vi "AlliGator Enter CV Analysis Parameters Dialog.vi"(8 "Error In":errorcluster) -> (0 "Error Out":errorcluster, 1 "Cancelled?":bool, 3 "Function Parameters out":T1={"Function"=enum."Single-Exponential", "Amplitude"=0.0, "Exponent/Scale"=0.0, "Baseline"=0.0, "Residuals SDV"=0.0, "Minimum CL (%)"=1.0, "Analysis Type"=enum."Reference", "Bootstrap SDV x Scale Factor"=1.0, "Residuals SDV x Scale Factor"=1.0, "Low CL Percentile to Reject (%)"=1.0} {"Low CL Percentile to Reject (%)" min=0.0 max=100.0; "Residuals SDV x Scale Factor" min=0.0 max=100.0; "Bootstrap SDV x Scale Factor" min=0.0 max=100.0; "Minimum CL (%)" min=1.0})   [LabVIEW 2021, in "AlliGator Decay Fit Parameter Map.lvlib"]
doc: "Lets the user enter the power law parameters describing the CV_tau(I) dependency, where <B>I</B> is the pixel intensity and <B>CV_tau</B> is the lifetime coefficient of variation obtained from calibration measurements."
uses:
  AlliGator Decay Fit Parameter Map.lvlib
  AlliGator Function Parameters.ctl
  AlliGator CV(tau) Model Function.ctl
  Lifetime & Other Parameters/AlliGator Lifetime & Other Parameters.lvlib
panel:
  in  "Function Parameters":T1={"Function"=enum."Single-Exponential", "Amplitude"=0.0, "Exponent/Scale"=0.0, "Baseline"=0.0, "Residuals SDV"=0.0, "Minimum CL (%)"=1.0, "Analysis Type"=enum."Reference", "Bootstrap SDV x Scale Factor"=1.0, "Residuals SDV x Scale Factor"=1.0, "Low CL Percentile to Reject (%)"=1.0} {"Low CL Percentile to Reject (%)" min=0.0 max=100.0; "Residuals SDV x Scale Factor" min=0.0 max=100.0; "Bootstrap SDV x Scale Factor" min=0.0 max=100.0; "Minimum CL (%)" min=0.0 max=100.0}
  out "Message":string
  in  "Cancel":bool
  in  "OK":bool
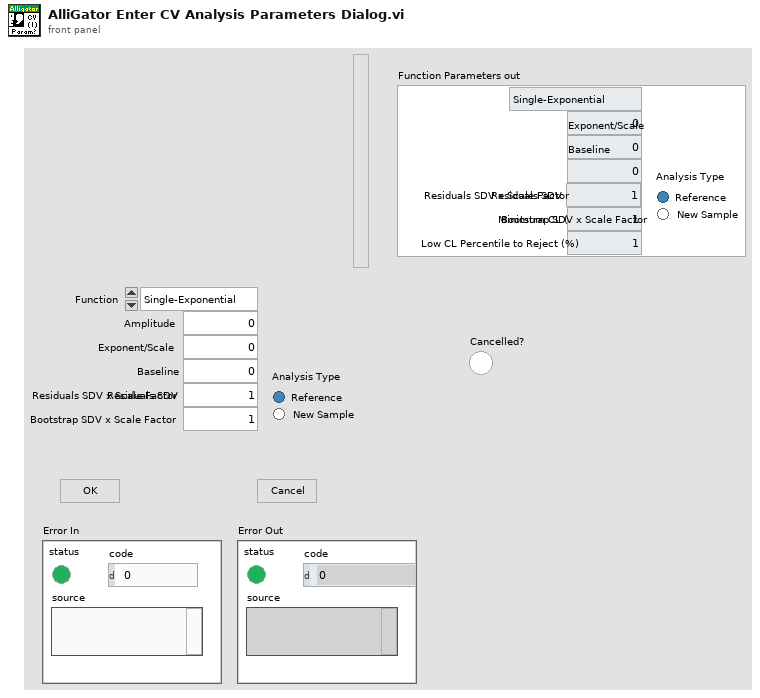
[diagram p1: front panel]
types:
  T1 = typedef "AlliGator Decay Fit Parameter Map.lvlib/AlliGator Function Parameters.ctl" = cluster{"Function":T2, "Amplitude":dbl, "Exponent/Scale":dbl, "Baseline":dbl, "Residuals SDV":dbl, "Minimum CL (%)":dbl, "Analysis Type":enum32{"Reference", "New Sample"}, "Bootstrap SDV x Scale Factor":dbl, "Residuals SDV x Scale Factor":dbl, "Low CL Percentile to Reject (%)":dbl}
  T2 = typedef "AlliGator Lifetime & Other Parameters.lvlib/AlliGator CV(tau) Model Function.ctl" = enum16{"Single-Exponential", "Power Law"}
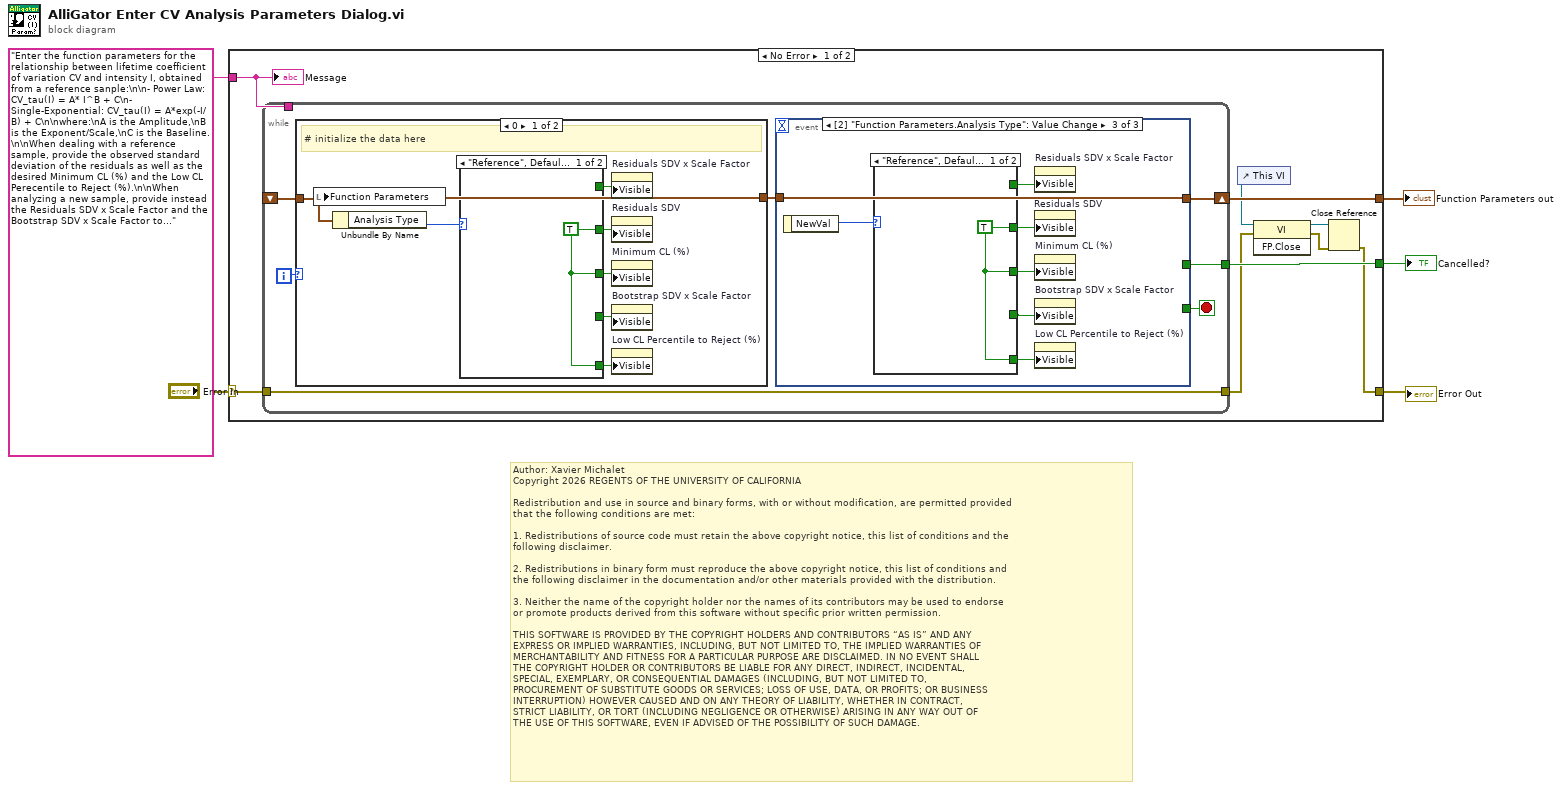
[diagram p0: block diagram]
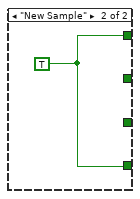
[diagram p2: hidden frame]
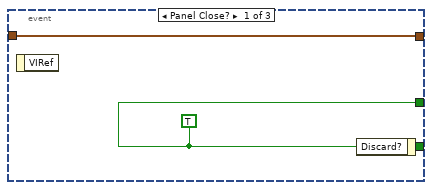
[diagram p4: hidden frame]
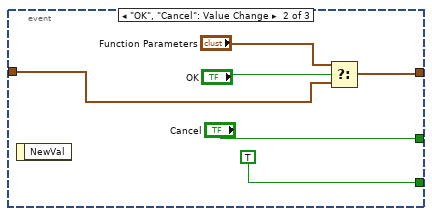
[diagram p5: hidden frame]
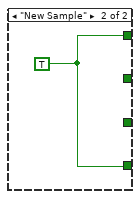
[diagram p6: hidden frame]
diagram:
  # "Author: Xavier Michalet\nCopyright 2026 REGENTS OF THE UNIVERSITY OF CALIFORNIA\n\nRedistribution and use in source and binary forms, with or without modification, are permitted provided\nthat the following conditions are met:\n\n1. Redistributions of source code must retain the above copyright notice, this list of conditions and the\nfollowing disclaimer.\n\n2. Redistributions in binary form must reproduce the above copyright notice, this list of conditions and\nthe following disclaimer in the documentation and/or other materials provided with the distribution.\n\n3. Neither the name of the copyright holder nor the names of its contributors may be used to endorse \nor promote products derived from this software without specific prior written permission.\n\nTHIS SOFTWARE IS PROVIDED BY THE COPYRIGHT HOLDERS AND CONTRIBUTORS “AS IS” AND ANY \nEXPRESS OR IMPLIED WARRANTIES, INCLUDING, BUT NOT LIMITED TO, THE IMPLIED WARRANTIES OF\nMERCHANTABILITY AND FITNESS FOR A PARTICULAR PURPOSE ARE DISCLAIMED. IN NO EVENT SHALL\nTHE COPYRIGHT HOLDER OR CONTRIBUTORS BE LIABLE FOR ANY DIRECT, INDIRECT, INCIDENTAL, \nSPECIAL, EXEMPLARY, OR CONSEQUENTIAL DAMAGES (INCLUDING, BUT NOT LIMITED TO, \nPROCUREMENT OF SUBSTITUTE GOODS OR SERVICES; LOSS OF USE, DATA, OR PROFITS; OR BUSINESS\nINTERRUPTION) HOWEVER CAUSED AND ON ANY THEORY OF LIABILITY, WHETHER IN CONTRACT, \nSTRICT LIABILITY, OR TORT (INCLUDING NEGLIGENCE OR OTHERWISE) ARISING IN ANY WAY OUT OF\nTHE USE OF THIS SOFTWARE, EVEN IF ADVISED OF THE POSSIBILITY OF SUCH DAMAGE."
  n1 = case shown="No Error" "Error In" {
    selector: "Error In" -> [w10 w49]
    tunnel: [w14 _] -> w5
    tunnel: [w13 _] -> w4
    tunnel: "Enter the function parameters for the relationship between lifetime coefficient of variation CV and intensity I, obtained from a reference sanple:\n\n- Power Law: CV_tau(I) = A* I^B + C\n- Single-Exponential: CV_tau(I) = A*exp(-I/B) + C\n\nwhere:\nA is the Amplitude,\nB is the Exponent/Scale,\nC is the Baseline.\n\nWhen dealing with a reference sample, provide the observed standard deviation of the residuals as well as the desired Minimum CL (%) and the Low CL Perecentile to Reject (%).\n\nWhen analyzing a new sample, provide instead the Residuals SDV x Scale Factor and the Bootstrap SDV x Scale Factor to use in order to compute the CL maps." ("Input Message") -> [w12 _]
    tunnel: [w11 w49] -> w2
    frame No Error {
      n2 = while {
        tunnel: [w20] -> w14
        shift-right: [w17] -> w13
        shift-left: _ -> [w18]
        tunnel: w12 -> [_]
        tunnel: w10 -> [w15]
        tunnel: [w15] -> w7
        i -> [w19]
        stop <- w21 stop-if-true
        n3 = case shown="0" w19 {
          tunnel: w18 -> [w28 w31]
          tunnel: [w28 w31] -> w16
          frame 0 {
            # "# initialize the data here"
            n4 = local write "Function Parameters"(w28) -> ()
            n5 = Unbundle By Name(w28) -> ("Analysis Type"=w27:enum32{"Reference", "New Sample"})
            n6 = case shown="\"Reference\", Default" w27 {
              tunnel: [_ w30] -> w26
              tunnel: [w29 _] -> w25
              tunnel: [w29 _] -> w24
              tunnel: [_ w30] -> w23
              tunnel: [w29 _] -> w22
              frame "Reference", Default {
                w29 = TRUE ("Visible")
              }
              frame "New Sample" {
                w30 = TRUE ("Visible")
              }
            }
            n7 = property on="Residuals SDV x Scale Factor" class="DigNum (strict)"("Visible"=w26) -> ()  [unwired: 2 in, 2 out]
            n8 = property on="Residuals SDV" class="DigNum (strict)"("Visible"=w25) -> ()  [unwired: 2 in, 2 out]
            n9 = property on="Minimum CL (%)" class="DigNum (strict)"("Visible"=w24) -> ()  [unwired: 2 in, 2 out]
            n10 = property on="Bootstrap SDV x Scale Factor" class="DigNum (strict)"("Visible"=w23) -> ()  [unwired: 2 in, 2 out]
            n11 = property on="Low CL Percentile to Reject (%)" class="DigNum (strict)"("Visible"=w22) -> ()  [unwired: 2 in, 2 out]
          }
          frame 1, Default {
          }
        }
        n12 = event shown="[2] \"Function Parameters.Analysis Type\": Value Change" {
          selector: _ -> [_ _ _]
          dyn-events: _ -> [_ _ _]
          timeout: _ -> [_ _ _]
          tunnel: [w33 TRUE ("Discard?") _] -> w21
          tunnel: [w33 "Cancel" _] -> w20
          tunnel: [w32 w35 w45] -> w17
          tunnel: w16 -> [w32 w34 w45]
          event Panel Close? {
            w33 = TRUE ("Discard?")
            n13 = event-data() -> ()  [unwired: 1 in, 1 out]
            n14 = event-data("Discard?"=w33) -> ()  [unwired: 1 in, 1 out]
          }
          event "OK", "Cancel": Value Change {
            n15 = event-data() -> ()  [unwired: 1 in, 1 out]
            n16 = Select(t="Function Parameters", s="OK", f=w34) -> (s? t:f=w35:T1)
          }
          event Value Change {
            n17 = event-data() -> ("NewVal"=w46:enum32{"Reference", "New Sample"})  [unwired: 1 in]
            n18 = case shown="\"Reference\", Default" w46 {
              tunnel: [_ w48] -> w44
              tunnel: [w47 _] -> w43
              tunnel: [w47 _] -> w42
              tunnel: [_ w48] -> w41
              tunnel: [w47 _] -> w40
              frame "Reference", Default {
                w47 = TRUE ("Visible")
              }
              frame "New Sample" {
                w48 = TRUE ("Visible")
              }
            }
            n19 = property on="Residuals SDV x Scale Factor" class="DigNum (strict)"("Visible"=w44) -> ()  [unwired: 2 in, 2 out]
            n20 = property on="Residuals SDV" class="DigNum (strict)"("Visible"=w43) -> ()  [unwired: 2 in, 2 out]
            n21 = property on="Minimum CL (%)" class="DigNum (strict)"("Visible"=w42) -> ()  [unwired: 2 in, 2 out]
            n22 = property on="Bootstrap SDV x Scale Factor" class="DigNum (strict)"("Visible"=w41) -> ()  [unwired: 2 in, 2 out]
            n23 = property on="Low CL Percentile to Reject (%)" class="DigNum (strict)"("Visible"=w40) -> ()  [unwired: 2 in, 2 out]
          }
        }
      }
      n24 = control-ref of="This VI"() -> (w6:refnum<vi>)
      n25 = invoke class="VI" method="FP.Close"(reference=w6, error in=w7) -> (reference out=w9:refnum<vi>, error out=w8:errorcluster)  [unwired: 1 in, 1 out]
      n26 = Close Reference(reference=w9, error in (no error)=w8) -> (error out=w11:errorcluster)
      "Message" <- w12
    }
    frame Error {
    }
  }
  "Function Parameters out" <- w4
  "Cancelled?" <- w5
  "Error Out" <- w2
